vi "fgt set Ttl Mode.vi"(8 "error in (no error)":errorcluster, 10 "mode":T1, 11 "TtlIndex":u32) -> (0 "error out":errorcluster)   [LabVIEW 2020, in "fgt_SDK.lvlib"]
doc: "Configure a specific TTL port (BNC ports) as input, output, rising or falling edge."
uses:
  fgt_SDK.lvlib
  TypeDefs/fgt_TTL_MODE.ctl
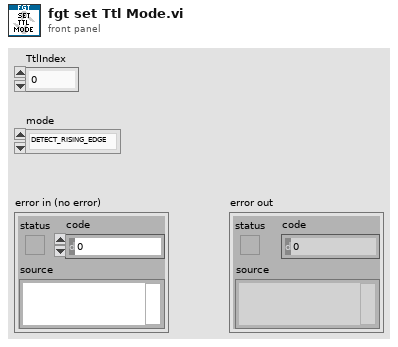
[diagram p1: front panel]
types:
  T1 = typedef "fgt_SDK.lvlib/fgt_TTL_MODE.ctl" = enum16{"DETECT_RISING_EDGE", "DETECT_FALLING_EDGE", "OUTPUT_PULSE_LOW", "OUTPUT_PULSE_HIGH"}
  T2 = typedef "fgt_SDK.lvlib/fgt_STATUS_INFO.ctl" = cluster{"InstrType":T3, "instrSN":u16, "errorCode":u8, "infoCode":u8, "detail":string}
  T3 = typedef "fgt_SDK.lvlib/fgt_INSTRUMENT_TYPE.ctl" = enum32{"None", "MFCS", "MFCS_EZ", "FRP", "LineUP", "IPS"}
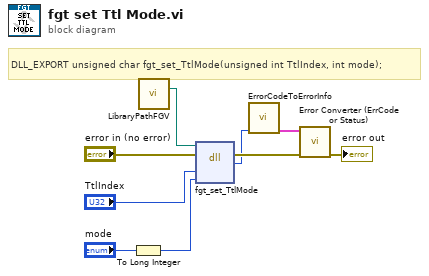
[diagram p0: block diagram]
diagram:
  # "DLL_EXPORT unsigned char fgt_set_TtlMode(unsigned int TtlIndex, int mode);"
  n1 = To Long Integer(number="mode") -> (32bit integer=w4:i32)
  n2 = call "LibraryPathFGV.vi"() -> ("Path Out"=w1:path)  [unwired: 14 in, 1 out]
  n3 = dll-call lib="C:/Workspace/fgt-SDK/LabVIEW/dlls/fgt_SDK_*.*" fn="fgt_set_TtlMode"(path in=w1, error in="error in (no error)", "TtlIndex"="TtlIndex", "mode"=w4) -> (error out=w6:errorcluster, "return type"=w3:u8)  [unwired: 3 in, 1 out]
  n4 = call "ErrorCodeToErrorInfo.vi"("return type"=w3) -> ("StatusInfo"=w2:T2)  [unwired: 10 in]
  n5 = call "Error Converter (ErrCode or Status).vi"("error in (no error)"=w6, "StatusInfo"=w2) -> ("error out"=→"error out":errorcluster)  [unwired: 9 in]
